vi "Olivetti_faces.vi"(8 "error in (no error)":errorcluster caption="entrée d'erreur (pas d'erreur)", 11 "fetch_olivetti_faces":T2={"shuffle"=FALSE, "random_state"=0, "download_if_missing"=TRUE, "Returns"="Data"} {"random_state" min=-1}) -> (0 "error out":errorcluster, 3 "Data":T1)   [LabVIEW 2020]
doc: "Labels associated to each face image. Those labels are ranging from 0-39 and correspond to the Subject IDs.\n\nThere are ten different images of each of 40 distinct subjects. For some subjects, the images were taken at different times, varying the lighting, facial expressions (open / closed eyes, smiling / not smiling) and facial details (glasses / no glasses). All the images were taken against a dark homogeneous background with the subjects in an upright, frontal position (with tolerance for some side movement).\n\nData Set Characteristics :\n - Classes : 40\n - Samples total : 400\n - Dimensionality : 4096\n - Features : real, between 0 and 1\n\nThe image is quantized to 256 grey levels and stored as unsigned 8-bit integers; the loader will convert these to floating point values on the interval [0, 1], which are easier to work with for many algorithms.\n\nThe “target” for this database is an integer from 0 to 39 indicating the identity of the person pictured; however, with only 10 examples per class, this relatively small dataset is more interesting from an unsupervised or semi-supervised perspective.\n\nThe original dataset consisted of 92 x 112, while the version available here consists of 64x64 images.\n\nWhen using these images, please give credit to AT&T Laboratories Cambridge.\n\nParameters : \n\n- shuffle : boolean, optional\nIf True the order of the dataset is shuffled to avoid having images of the same person grouped.\n\n- random_state : int, RandomState instance or None=-1, default=0\nDetermines random number generation for dataset shuffling. Pass an int for reproducible output across multiple function calls. See Glossary.\n\n- download_if_missing : optional, True by default\nIf False, raise a IOError if the data is not locally available instead of trying to download the data from the source site.\n\n\nReturns :\n\n- data : ndarray, shape (400, 64, 64)\nEach row is a face image corresponding to one of the 40 subjects of the dataset.\n\n- target : ndarray, shape (400,)"
uses:
  Olivetti_faces.lvclass
panel:
  out "Olivetti_faces.lvclass":refnum<class "Olivetti_faces.lvclass">
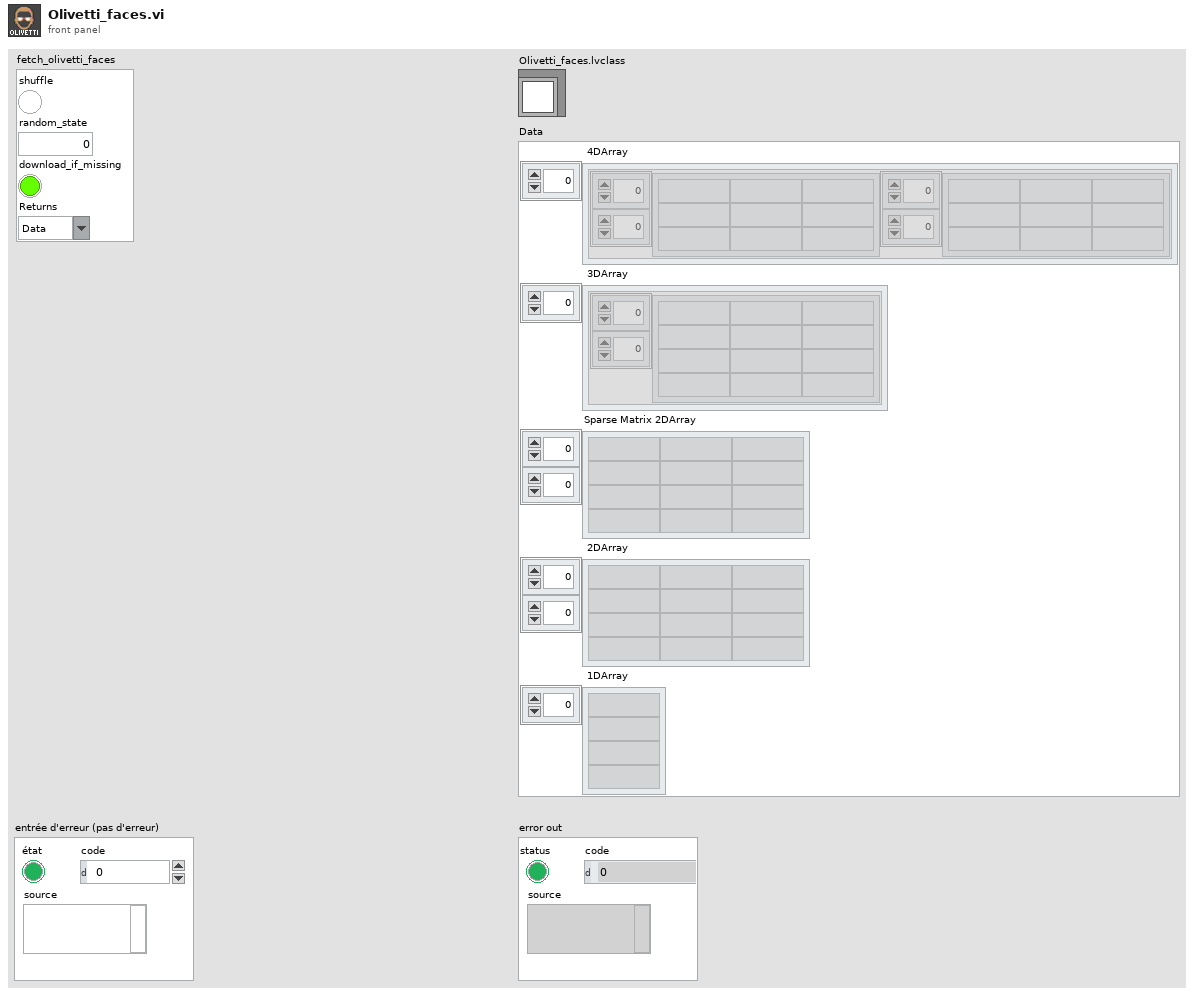
[diagram p1: front panel]
types:
  T1 = cluster{" 4DArray":cluster{"1":string[][], "2":string[][]}[], " 3DArray":cluster{"Tableau":string[][]}[], "Sparse Matrix 2DArray":string[][], " 2DArray":string[][], " 1DArray":string[]}
  T2 = cluster{"shuffle":bool, "random_state":i32, "download_if_missing":bool, "Returns":string}
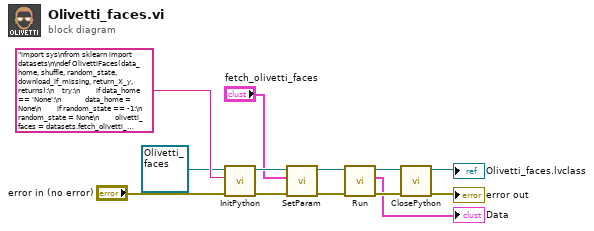
[diagram p0: block diagram]
diagram:
  n1 = call-dynamic "InitPython.vi"("error in (no error)"="error in (no error)", "Python Instruction"="import sys\nfrom sklearn import datasets\n\ndef OlivettiFaces(data_home, shuffle, random_state, download_if_missing, return_X_y, returns):\n    try:\n        if data_home == 'None':\n            data_home = None\n        if random_state == -1:\n            random_state = None\n        olivetti_faces = datasets.fetch_olivetti_faces(data_home, shuffle, random_state, download_if_missing, return_X_y)\n        if returns == 'Data':\n            data = olivetti_faces['images'].tolist()\n            return str(data)\n        else :\n            data = olivetti_faces['target'].tolist()\n            return str(data)  \n    except:\n        erreur = sys.exc_info()\n        typerr = u\"%s\" % (erreur[0])\n        typerr = typerr[typerr.find(\"'\")+1:typerr.rfind(\"'\")]\n        msgerr = u\"%s\" % (erreur[1])\n        message = str('/!\\\\ {0} : {1}'. format(typerr,msgerr))\n        return message", "Scikit-learn en entrée"=refnum<class "Olivetti_faces.lvclass"> refnum ("Olivetti_faces.lvclass")) -> ("error out"=w6:errorcluster, "Scikit-learn en sortie"=w8:refnum<class "Olivetti_faces.lvclass">)  [unwired: 7 in]
  n2 = call-dynamic "SetParam.vi"("error in (no error)"=w6, "fetch_olivetti_faces"="fetch_olivetti_faces", "Olivetti_faces.lvclass"=w8) -> ("error out"=w4:errorcluster, "Olivetti_faces.lvclass"=w5:refnum<class "Olivetti_faces.lvclass">)  [unwired: 7 in]
  n3 = call-dynamic "Run.vi"("error in (no error)"=w4, "Olivetti_faces.lvclass"=w5) -> ("error out"=w10:errorcluster, "Data"=→"Data":T1, "Olivetti_faces.lvclass"=w9:refnum<class "Olivetti_faces.lvclass">)  [unwired: 7 in]
  n4 = call-dynamic "ClosePython.vi"("error in (no error)"=w10, "Scikit-learn en entrée"=w9) -> ("error out"=→"error out":errorcluster, "Scikit-learn en sortie"=→"Olivetti_faces.lvclass":refnum<class "Olivetti_faces.lvclass">)  [unwired: 8 in]
